vi "MCB2300 PWM ProjectAttrValidator.vi"(5 "Ctl Refnum":refnum<vi>, 9 "PWMNum (0-6)":u8(ring) items=["9", "10", "11", "12", "13", "14", "15"], 11 "Attributes":T1={"Offset%"=50, "Double edge?"=FALSE, "Polarity"=FALSE, "Frequency (Hz)"=1000, "Programmable Pin Connections"=0} {"Programmable Pin Connections" items=["PWM1 and LED0 use pin P2.0. You cannot use PWM1 and LED0 in the same project.", "PWM2 and LED1 use pin P2.1. You cannot use PWM2 and LED1 in the same project.", "PWM3 and LED2 use pin P2.2. You cannot use PWM3 and LED2 in the same project.", "PWM4 and LED3 use pin P2.3. You cannot use PWM4 and LED3 in the same project.", "PWM5 and LED4 use pin P2.4. You cannot use PWM5 and LED4 in the same project.", "PWM6 and LED5 use pin P2.5. You cannot use PWM6 and LED5 in the same project."]}) -> (3 "Valid?":bool)   [LabVIEW 2011]
uses:
  <vilib>/Embedded/ARM/MCB2300/MCB2300_PWM_PrjAttr.ctl
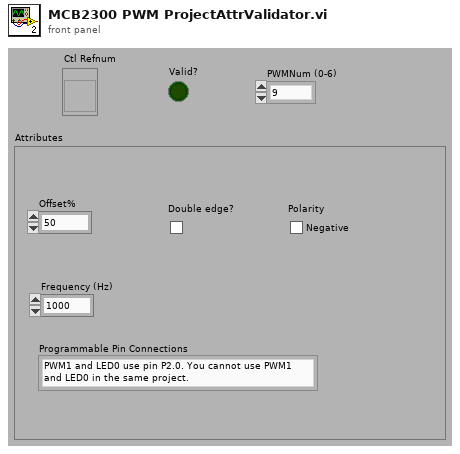
[diagram p1: front panel]
types:
  T1 = typedef "MCB2300_PWM_PrjAttr.ctl" = cluster{"Offset%":u8, "Double edge?":bool, "Polarity":bool, "Frequency (Hz)":u32, "Programmable Pin Connections":u16}
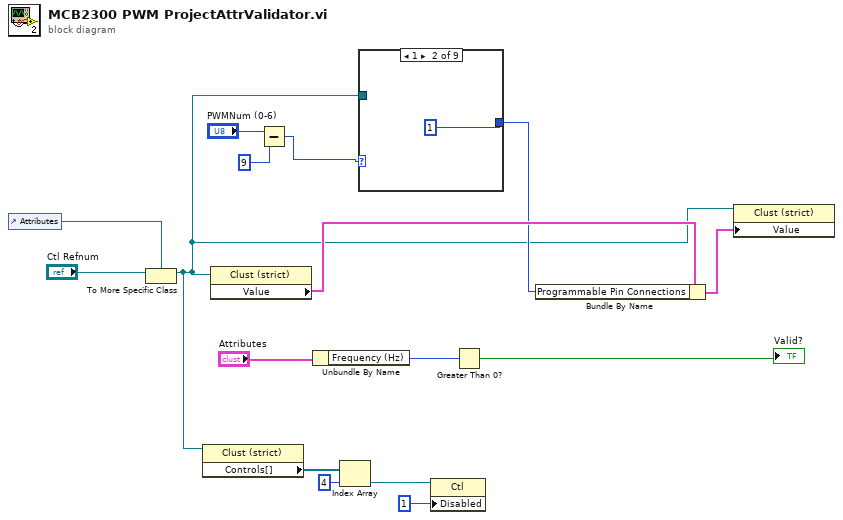
[diagram p0: block diagram]
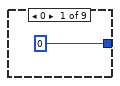
[diagram p2: hidden frame]
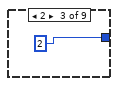
[diagram p3: hidden frame]
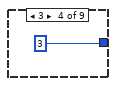
[diagram p4: hidden frame]
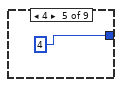
[diagram p5: hidden frame]
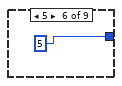
[diagram p6: hidden frame]
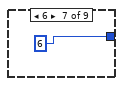
[diagram p7: hidden frame]
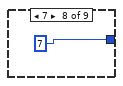
[diagram p8: hidden frame]
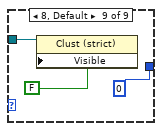
[diagram p9: hidden frame]
diagram:
  n1 = control-ref of="Attributes"() -> (w1:refnum<vi>)
  n2 = To More Specific Class(target class=w1, reference="Ctl Refnum") -> (specific class reference=w5:refnum<vi>)  [unwired: 1 in, 1 out]
  n3 = property class="Clust (strict)"(reference=w5) -> ("Controls[]"=w13:refnum<vi>[])  [unwired: 1 in, 2 out]
  n4 = property class="Clust (strict)"(reference=w5) -> ("Value"=w15:T1)  [unwired: 1 in, 2 out]
  n5 = Subtract(x="PWMNum (0-6)", y=u32 9) -> (x-y=w4:u32)
  n6 = Unbundle By Name("Attributes") -> ("Frequency (Hz)"=w9:u32)
  n7 = Index Array(array=w13, index=4) -> (element=w11:refnum<vi>)
  n8 = case shown="1" w4 {
    tunnel: [0 1 2 3 4 5 6 7 0] -> w7
    tunnel: w5 -> [_ _ _ _ _ _ _ _ w25]
    frame 0 {
    }
    frame 1 {
    }
    frame 2 {
    }
    frame 3 {
    }
    frame 4 {
    }
    frame 5 {
    }
    frame 6 {
    }
    frame 7 {
    }
    frame 8, Default {
      n9 = property class="Clust (strict)"(reference=w25, "Visible"=FALSE) -> ()  [unwired: 1 in, 2 out]
    }
  }
  n10 = property class="Ctl"(reference=w11, "Disabled"=u8 1) -> ()  [unwired: 1 in, 2 out]
  n11 = Greater Than 0?(x=w9) -> (x > 0?=→"Valid?":bool)
  n12 = Bundle By Name(cluster=w15, "Programmable Pin Connections"=w7) -> (w14:T1)
  n13 = property class="Clust (strict)"(reference=w5, "Value"=w14) -> ()  [unwired: 1 in, 2 out]
